vi "ma_SML Averaging (real input).vi"(3 "reset?":bool, 4 "averaging settings":T1, 5 "x":dbl[](array[numeric]) format="%.2f") -> (0 "data ready?":bool, 1 "averaged sofar":dbl, 2 "y":dbl[](array[numeric]) format="%.2f")   [LabVIEW 2020, in "NI_MAPro.lvlib"]
uses:
  NI_MAPro.lvlib
  ma_sml_Averaging Settings.ctl
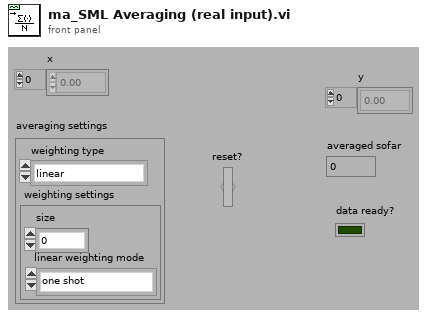
[diagram p1: front panel]
types:
  T1 = typedef "NI_MAPro.lvlib/ma_sml_Averaging Settings.ctl" = cluster{"weighting type":enum16{"linear", "exponential"}, "weighting settings":cluster{"size":dbl, "linear weighting mode":enum16{"one shot", "auto restart one shot", "moving average", "continuous"}}}
  T2 = cluster{"size":dbl, "linear weighting mode":enum16{"one shot", "auto restart one shot", "moving average", "continuous"}}
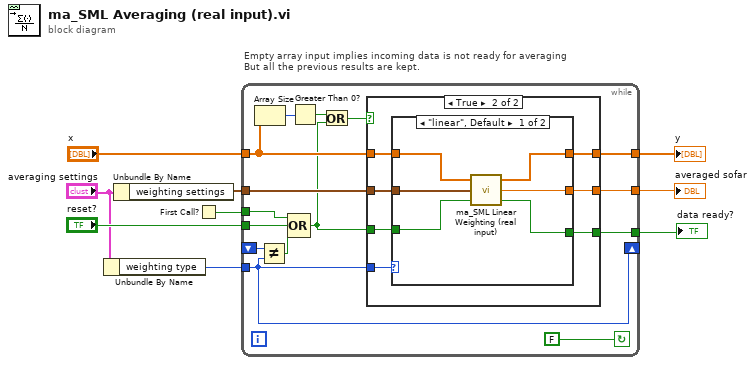
[diagram p0: block diagram]
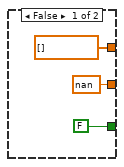
[diagram p2: hidden frame]
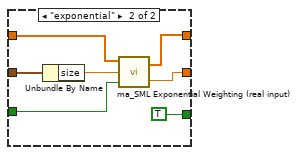
[diagram p3: hidden frame]
diagram:
  # "Empty array input implies incoming data is not ready for averaging\nBut all the previous results are kept."
  n1 = Unbundle By Name("averaging settings") -> ("weighting type"=w3:enum16{"linear", "exponential"})
  n2 = Unbundle By Name("averaging settings") -> ("weighting settings"=w2:T2)
  n3 = First Call?() -> (First Call?: T/F=w1:bool)
  n4 = while {
    tunnel: w1 -> [w10]
    shift-left: _ -> [w18]
    shift-right: [w19] -> _
    tunnel: w2 -> [w21]
    tunnel: w3 -> [w19]
    tunnel: [w22] -> w5
    tunnel: [w23] -> w6
    tunnel: "x" -> [w15]
    tunnel: "reset?" -> [w20]
    tunnel: [w24] -> w9
    stop <- FALSE continue-if-true
    n5 = Array Size(array=w15) -> (size(s)=w14:i32)
    n6 = Not Equal?(x=w18, y=w19) -> (x != y?=w17:bool)
    n7 = Compound Arithmetic op=OR(w10, w20, w17) -> (w11:bool)
    n8 = Greater Than 0?(x=w14) -> (x > 0?=w13:bool)
    n9 = Or(x=w13, y=w11) -> (x .or. y?=w12:bool)
    n10 = case shown="True" w12 {
      tunnel: [dbl[] [] ("y") w34] -> w24
      tunnel: w15 -> [_ w33]
      tunnel: [nan ("Average So-far") w32] -> w23
      tunnel: [FALSE ("DataReady") w31] -> w22
      tunnel: w21 -> [_ w30]
      tunnel: w11 -> [_ w29]
      tunnel: w19 -> [_ w28]
      frame False {
      }
      frame True {
        n11 = case shown="\"linear\", Default" w28 {
          tunnel: w30 -> [w40 w47]
          tunnel: w29 -> [w39 w44]
          tunnel: [w38 w43] -> w34
          tunnel: w33 -> [w37 w45]
          tunnel: [w36 w42] -> w32
          tunnel: [w35 TRUE ("DataReady")] -> w31
          frame "linear", Default {
            n12 = call "ma_SML Linear Weighting (real input).vi"("reset?"=w39, "settings"=w40, "x"=w37) -> ("data ready?"=w35:bool, "averaged sofar"=w36:dbl, "y"=w38:dbl[])
          }
          frame "exponential" {
            n13 = Unbundle By Name(w47) -> ("size"=w46:dbl)
            n14 = call "ma_SML Exponential Weighting (real input).vi"("reset?"=w44, "average size"=w46, "x"=w45) -> ("averaged sofar"=w42:dbl, "y"=w43:dbl[])
          }
        }
      }
    }
  }
  "y" <- w9
  "averaged sofar" <- w6
  "data ready?" <- w5
